vi "Edit-measurement-settings.vi"(8 "error in (no error)":errorcluster, 11 "Object ref in":T1) -> (0 "error out":errorcluster, 3 "Object ref out":T1)   [LabVIEW 2013, in "HardwareCharacterization.lvlib" / "HC-Main.lvclass"]
uses:
  HC-Main.lvclass
  Object-reference.ctl
  HC-Main.lvclass/HC-Main.ctl
  Read Measurement type.vi
  Read Parser.vi
  Read SM1000.vi
  Read LaserResponse.vi
  ScanParser/HC-ScanParser.lvclass
  SM1000/HC-SM1000.lvclass
  LaserPulseAnalyser/HC-LaserResponse.lvclass
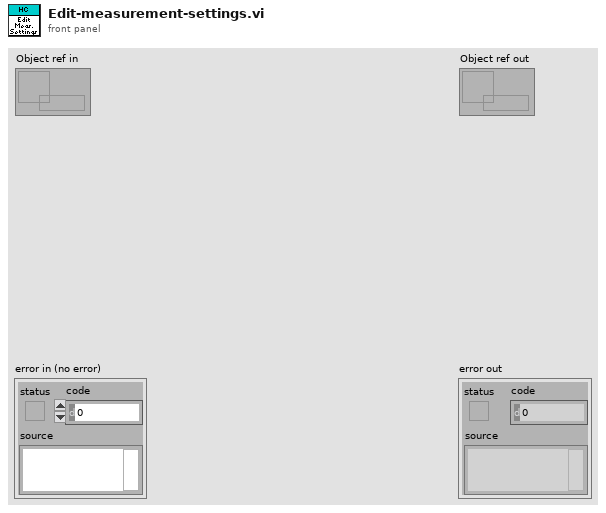
[diagram p1: front panel]
types:
  T1 = typedef "HardwareCharacterization.lvlib/HC-Main.lvclass/Object-reference.ctl" = refnum<data-value>
  T2 = typedef "HardwareCharacterization.lvlib/HC-Main.lvclass/Measurement-types.ctl" = enum16{"Scan file analysis", "SM1000 position conversion", "SM1000 modulation timing", "Laser output response"}
  T3 = typedef "HardwareCharacterization.lvlib/HC-ScanParser.lvclass/Object-reference.ctl" = refnum<data-value>
  T4 = typedef "HardwareCharacterization.lvlib/HC-SM1000.lvclass/Object-reference.ctl" = refnum<data-value>
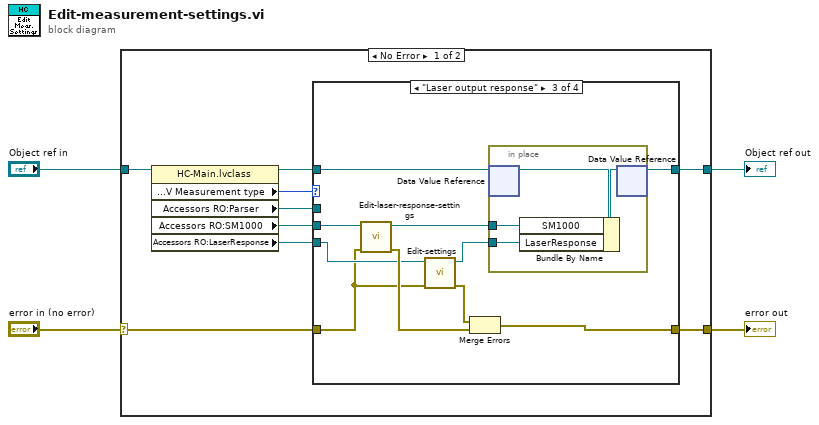
[diagram p0: block diagram]
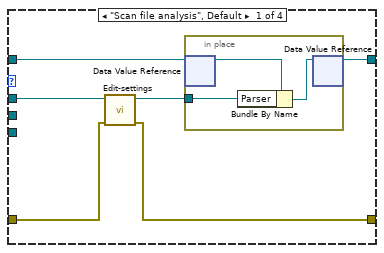
[diagram p2: hidden frame]
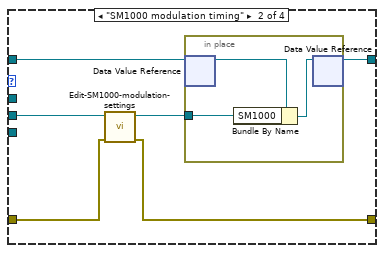
[diagram p3: hidden frame]
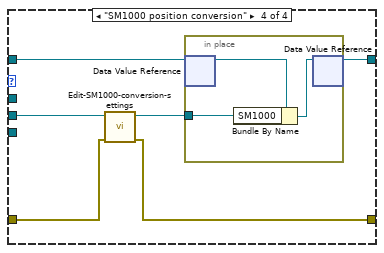
[diagram p4: hidden frame]
diagram:
  n1 = case shown="No Error" "error in (no error)" {
    selector: "error in (no error)" -> [w9 w56]
    tunnel: [w8 w56] -> w3
    tunnel: [w10 w55] -> w1
    tunnel: "Object ref in" -> [w13 w55]
    frame No Error {
      n2 = property class="HC-Main.lvclass"(reference=w13) -> (reference out=w11:T1, "Accessors/Modifiers:V Measurement type"=w12:T2, "Accessors RO:Parser"=w7:T3, "Accessors RO:SM1000"=w6:T4, "Accessors RO:LaserResponse"=w5:refnum<class "HC-LaserResponse.lvclass">)  [unwired: 1 in, 1 out]
      n3 = case shown="\"Laser output response\"" w12 {
        tunnel: w11 -> [w18 w28 w41 w51]
        tunnel: [w17 w27 w40 w50] -> w10
        tunnel: w9 -> [w15 w25 w34 w48]
        tunnel: [w14 w24 w33 w47] -> w8
        tunnel: w7 -> [w19 _ _ _]
        tunnel: w6 -> [_ w23 w37 w46]
        tunnel: w5 -> [_ _ w36 _]
        frame "Scan file analysis", Default {
          n4 = call "Edit-settings.vi"("error in (no error)"=w15, "Reference in"=w19) -> ("error out"=w14:errorcluster, "Reference out"=w16:T3)  [unwired: 8 in]
          n5 = in-place {
            in-place-border: w16 -> [w20]
            n6 = in-place-dvr #1(w18) -> (w22:refnum<class "HC-Main.lvclass">)  [unwired: 1 out]
            n7 = Bundle By Name(cluster=w22, "Parser"=w20) -> (w21:refnum<class "HC-Main.lvclass">)
            n8 = in-place-dvr #1(w21) -> (w17:T1)  [unwired: 1 out]
          }
        }
        frame "SM1000 modulation timing" {
          n9 = call "Edit-SM1000-modulation-settings.vi"("error in (no error)"=w25, "Reference in"=w23) -> ("error out"=w24:errorcluster, "Reference out"=w26:T4)  [unwired: 8 in]
          n10 = in-place {
            in-place-border: w26 -> [w29]
            n11 = in-place-dvr #2(w28) -> (w31:refnum<class "HC-Main.lvclass">)  [unwired: 1 out]
            n12 = Bundle By Name(cluster=w31, "SM1000"=w29) -> (w30:refnum<class "HC-Main.lvclass">)
            n13 = in-place-dvr #2(w30) -> (w27:T1)  [unwired: 1 out]
          }
        }
        frame "Laser output response" {
          n14 = call "Edit-laser-response-settings.vi"("error in (no error)"=w34, "Reference in"=w37) -> ("error out"=w38:errorcluster, "Reference out"=w39:T4)  [unwired: 8 in]
          n15 = call "Edit-settings.vi"("error in (no error)"=w34, "HC-LaserPulse in"=w36) -> ("error out"=w32:errorcluster, "HC-LaserPulse out"=w35:refnum<class "HC-LaserResponse.lvclass">)  [unwired: 8 in]
          n16 = Merge Errors(w32, w38) -> (w33:errorcluster)
          n17 = in-place {
            in-place-border: w39 -> [w43]
            in-place-border: w35 -> [w42]
            n18 = in-place-dvr #3(w41) -> (w45:refnum<class "HC-Main.lvclass">)  [unwired: 1 out]
            n19 = Bundle By Name(cluster=w45, "SM1000"=w43, "LaserResponse"=w42) -> (w44:refnum<class "HC-Main.lvclass">)
            n20 = in-place-dvr #3(w44) -> (w40:T1)  [unwired: 1 out]
          }
        }
        frame "SM1000 position conversion" {
          n21 = call "Edit-SM1000-conversion-settings.vi"("error in (no error)"=w48, "Reference in"=w46) -> ("error out"=w47:errorcluster, "Reference out"=w49:T4)  [unwired: 8 in]
          n22 = in-place {
            in-place-border: w49 -> [w52]
            n23 = in-place-dvr #4(w51) -> (w54:refnum<class "HC-Main.lvclass">)  [unwired: 1 out]
            n24 = Bundle By Name(cluster=w54, "SM1000"=w52) -> (w53:refnum<class "HC-Main.lvclass">)
            n25 = in-place-dvr #4(w53) -> (w50:T1)  [unwired: 1 out]
          }
        }
      }
    }
    frame Error {
    }
  }
  "error out" <- w3
  "Object ref out" <- w1
